vi "SellStock.vi"(8 "error in (no error)":errorcluster, 10 "Stock.lvclass":refnum<class "Stock.lvclass">, 11 "SellStock in":refnum<class "SellStock.lvclass">) -> (0 "error out":errorcluster, 3 "SellStock out":refnum<class "SellStock.lvclass">)   [LabVIEW 2017, in "SellStock.lvclass"]
uses:
  SellStock.lvclass
  Stock Class/Stock.lvclass
  SellStock.lvclass/SellStock.ctl
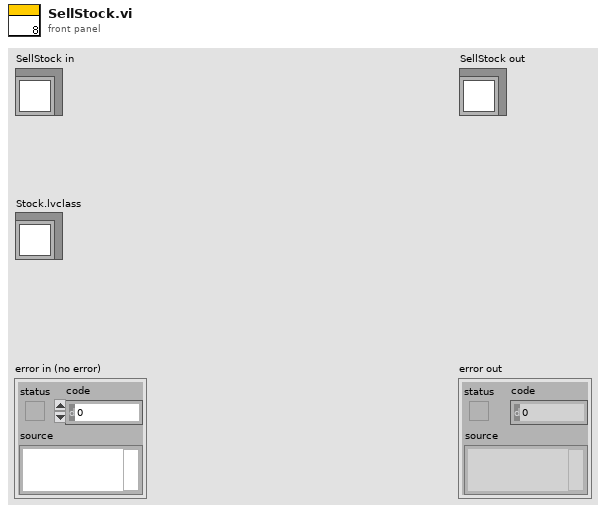
[diagram p1: front panel]
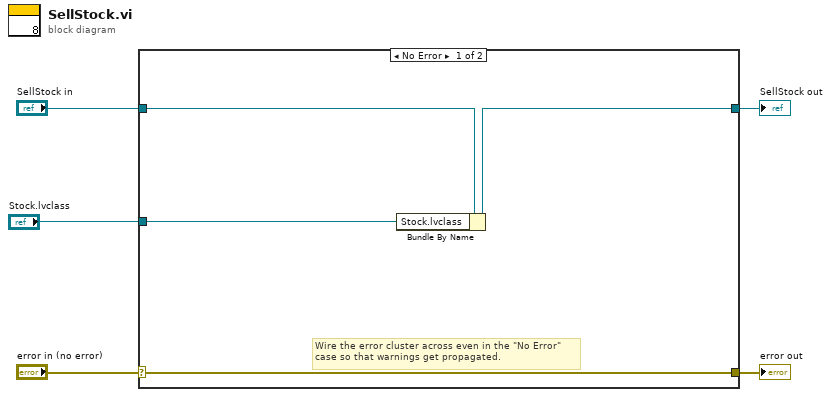
[diagram p0: block diagram]
diagram:
  n1 = case shown="No Error" "error in (no error)" {
    selector: "error in (no error)" -> [w8 w11]
    tunnel: [w8 w11] -> w4
    tunnel: [w7 w10] -> w2
    tunnel: "SellStock in" -> [w9 w10]
    tunnel: "Stock.lvclass" -> [w6 _]
    frame No Error {
      # "Wire the error cluster across even in the \"No Error\"\ncase so that warnings get propagated."
      n2 = Bundle By Name(cluster=w9, "Stock.lvclass"=w6) -> (w7:refnum<class "SellStock.lvclass">)
    }
    frame Error {
    }
  }
  "error out" <- w4
  "SellStock out" <- w2
